vi "Serial.vi"() -> ()   [LabVIEW 2019]
uses:
  <vilib>/Instr/_visa.llb/VISA Configure Serial Port (Instr).vi
panel:
  out "return count":u32
  out "Sequence No":string
  out "Data":string
  in  "stop":bool
  in  "VISA resource name":refnum<visa-resource-name>
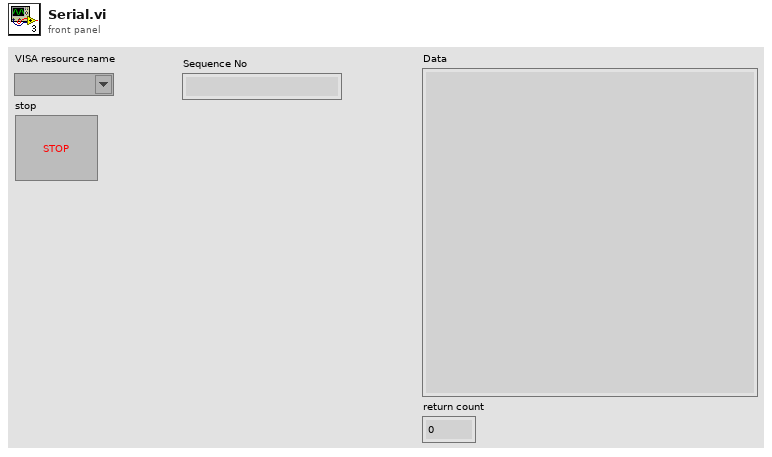
[diagram p1: front panel]
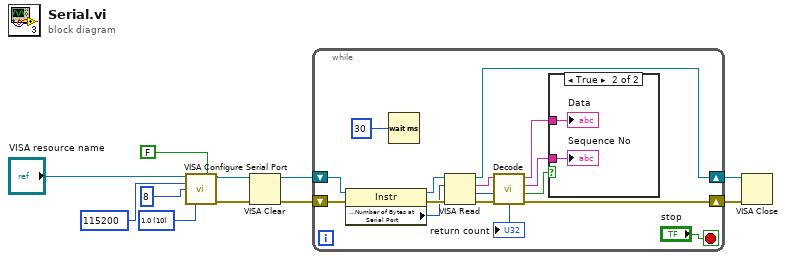
[diagram p0: block diagram]
diagram:
  w8 = u16 10 items=["1.0"=10, "1.5"=15, "2.0"=20] ("stop bits (10: 1 bit)")
  n1 = call-poly "VISA Configure Serial Port"("VISA resource name"="VISA resource name", "Enable Termination\nChar (T)"=FALSE ("Enable Termination\nChar (T)"), "baud rate (9600)"=u32 115200, "data bits (8)"=u16 8, "stop bits (10: 1 bit)"=w8) -> ("VISA resource name out"=w2:refnum<visa-resource-name>, "error out"=w4:errorcluster)  [unwired: 9 in]
  n2 = VISA Clear(VISA resource name=w2, error in (no error)=w4) -> (VISA resource name out=w1:refnum<visa-resource-name>, error out=w3:errorcluster)
  n3 = while {
    shift-right: [w26] -> w5
    shift-left: w1 -> [w15]
    shift-right: [w24] -> w6
    shift-left: w3 -> [w18]
    stop <- "stop" stop-if-true
    n4 = property class="Instr"(reference=w15, error in=w18) -> (reference out=w14:refnum<visa-resource-name>, error out=w17:errorcluster, "Serial Settings:Number of Bytes at Serial Port"=w16:u32)
    n5 = Wait (ms)(milliseconds to wait=u32 30) -> ()  [unwired: 1 out]
    n6 = VISA Read(VISA resource name=w14, byte count=w16, error in (no error)=w17) -> (VISA resource name out=w26:refnum<visa-resource-name>, read buffer=w22:string, return count=→"return count":u32, error out=w25:errorcluster)
    n7 = call "Decode.vi"("error in (no error)"=w25, "Raw Data"=w22) -> ("error out"=w24:errorcluster, "Success"=w21:bool, "Sequence No"=w19:string, "Data"=w20:string)  [unwired: 6 in]
    n8 = case shown="True" w21 {
      tunnel: w20 -> [_ w28]
      tunnel: w19 -> [_ w27]
      frame False {
      }
      frame True {
        "Data" <- w28
        "Sequence No" <- w27
      }
    }
  }
  n9 = VISA Close(VISA resource name=w5, error in (no error)=w6) -> ()  [unwired: 1 out]
